vi "Check Target Support.vi"(8 "error in":errorcluster, 11 "configuration in":refnum<class "TBM configuration.lvclass">) -> (0 "error out":errorcluster, 3 "configuration out":refnum<class "TBM configuration.lvclass">)   [LabVIEW 2013, in "TBM configuration.lvclass"]
doc: "This method uses the current operating system as well as support information provided by a specific configuration to determine if the current target is supported."
uses:
  TBM configuration.lvclass
  Target Types.ctl
  <vilib>/NI/Configuration Framework/NISE_CEF_TreeControl.lvlib
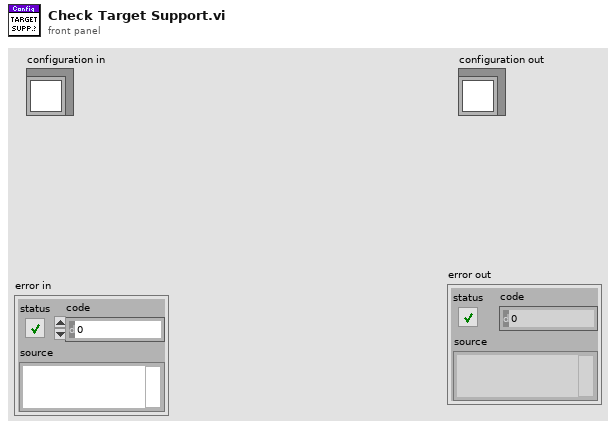
[diagram p1: front panel]
types:
  T1 = typedef "TBM configuration.lvclass/Target Types.ctl" = enum16{"Windows", "Mac", "Linux", "Linux RT ARM", "VxWorks", "Pharlap", "Other", "Linux RT x64"}
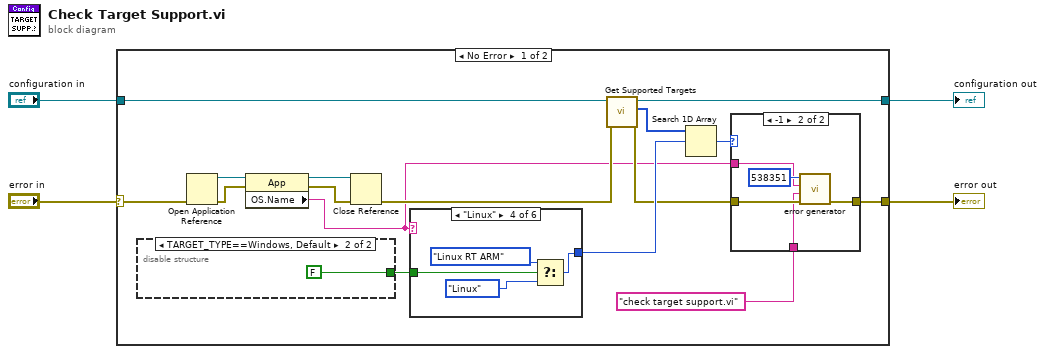
[diagram p0: block diagram]
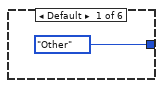
[diagram p3: hidden frame]
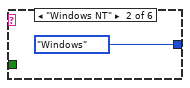
[diagram p4: hidden frame]
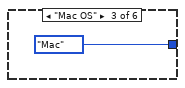
[diagram p5: hidden frame]
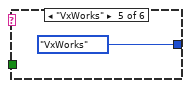
[diagram p6: hidden frame]
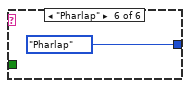
[diagram p7: hidden frame]
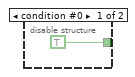
[diagram p8: hidden frame]
diagram:
  n1 = case shown="No Error" "error in" {
    selector: "error in" -> [w10 w38]
    tunnel: "configuration in" -> [w15 w39]
    tunnel: [w13 w39] -> w3
    tunnel: [w7 w38] -> w2
    frame No Error {
      n2 = disable-structure shown="TARGET_TYPE==Windows, Default" {
        disable-tunnel: [TRUE FALSE] -> w16
        frame condition #0 {
        }
        frame condition #1 (active) {
        }
      }
      n3 = Open Application Reference(8:w10) -> (0:w19:errorcluster, 3:w20:refnum<vi>)  [unwired: 3 in]
      n4 = property class="App"(reference=w20, error in=w19) -> (reference out=w18:refnum<vi>, error out=w17:errorcluster, "OS.Name"=w5:string)
      n5 = Close Reference(reference=w18, error in (no error)=w17) -> (error out=w11:errorcluster)
      n6 = case shown="\"Linux\"" w5 {
        tunnel: w16 -> [_ _ _ w33 _ _]
        tunnel: [Target_Types."Other" ("Target Types") Target_Types."Windows" ("Target Types") Target_Types."Mac" ("Target Types") w30 Target_Types."VxWorks" ("Target Types") Target_Types."Pharlap" ("Target Types")] -> w12
        frame Default {
        }
        frame "Windows NT" {
        }
        frame "Mac OS" {
        }
        frame "Linux" {
          n7 = Select(t=Target_Types."Linux RT ARM" ("Target Types"), s=w33, f=Target_Types."Linux" ("Target Types")) -> (s? t:f=w30:T1)
        }
        frame "VxWorks" {
        }
        frame "Pharlap" {
        }
      }
      n8 = call-dynamic "Get Supported Targets.vi"("error in"=w11, "configuration in"=w15) -> ("error out"=w8:errorcluster, "supported targets"=w14:T1[], "configuration out"=w13:refnum<class "TBM configuration.lvclass">)  [unwired: 7 in]
      n9 = Search 1D Array(1D array=w14, element=w12) -> (index of element=w9:i32)  [unwired: 1 in]
      n10 = case shown="-1" w9 {
        tunnel: w8 -> [w21 w25]
        tunnel: [w21 w26] -> w7
        tunnel: "check target support.vi" -> [_ w23]
        tunnel: w5 -> [_ w22]
        frame 0, Default {
        }
        frame -1 {
          n11 = call <vilib>:"error generator.vi"("error in"=w25, "source"=w23, "append error message"=w22, "error code (0)"=538351) -> ("error out"=w26:errorcluster)  [unwired: 5 in]
        }
      }
    }
    frame Error {
    }
  }
  "configuration out" <- w3
  "error out" <- w2
